vi "Goalie.vi"(3 "Defensores":u32[](array[numeric]), 5 "AI Parameters":T1={"GotoKick"={"Dist do cone a frente"=150.0, "attacker farback"=1500.0, "Perto"=300.0, "min dist to kick"=150.0, "kick eps"=0.0, "Time to transition"=0.05}, "Attacker"={"CC chute"=0.09, "CC passe"=0.045, "Kick Force"=100.0, "D ball-robot Kick"=200.0, "D ball-robot Pass"=0.3}, "Defender"={"D max"=1700.0, "Vel p/ robô av"=1000.0, "Kick Force"=100.0, "D atk-def"=0.0, "D farback"=0.0}, "Timeout"={"Field/v in x"=6.0, "Dist Robots"=300, "Dist up in y"=300}, "Pose Striker"={"dist"=200.0, "Numeric"=-4.0, "dist 2"=200.0}, "Dist Stop"=300.0, "Distance when ball out"=200, "D central gap "=150.0, "T pass"=0.0, "Force ++"=0.0, "range kick"=0.0, "Chute alto"=TRUE, "Marcador novo"=TRUE} {"D central gap" format="%#_13g"; "Dist Stop" format="%#_13g"; "Pose Striker"."Numeric" format="%#_13g"; "Defender"."Kick Force" format="%#_13g"; "Defender"."Vel p/ robô av" format="%#_13g"; "Attacker"."D ball-robot Kick" format="%#_13g"; "Attacker"."Kick Force" format="%#_13g"; "Attacker"."CC passe" format="%#_13g"; "Attacker"."CC chute" format="%#_13g"; "GotoKick"."kick eps" format="%#_13g"; "GotoKick"."min dist to kick" format="%#_13g"; "GotoKick"."Perto" format="%#_13g"; "GotoKick"."attacker farback" format="%#_13g"; "GotoKick"."Dist do cone a frente" format="%#_13g"}, 7 "Total de robos":u32[](array[numeric]), 8 "Field defense":dbl[](array[numeric]), 9 "IA Input":T5={"our_robots"=[], "enemy_robots"=[], "balls"=[], "geometry"={"line_width"=0, "field_length"=0, "field_width"=0, "boundary_width"=0, "referee_width"=0, "goal_width"=0, "goal_depth"=0, "goal_wall_width"=0, "center_circle_radius"=0, "defense_radius"=0, "defense_stretch"=0, "free_kick_from_defense_dist"=0, "penalty_spot_from_field_line_dist"=0, "penalty_line_from_spot_dist"=0}, "IA Judge"={"stage"="", "command"="", "our_goalie_id"=0.0, "enemy_goalie_id"=0.0, "command enum"=enum."Halt", "Time"=enum."Azul"}, "Received Timestamp"=timestamp(0 s since 1904-01-01), "Events"={"Touch"=FALSE, "Ball out"=FALSE, "id touch"=0.0, "Ball out of \nVision"=FALSE, "Ball inside \nGoalie area"=FALSE, "Robot not responding"=FALSE, "Robots responding status"=[1.0, 1.0, 1.0, 1.0, 1.0, 1.0], "Enemy Ball \nPossession"=FALSE, "Pass State"=FALSE, "id end of pass"=0.0, "Kick"=FALSE, "Id ini Possession"=0.0, "Ball Possesion"=FALSE, "Id Possesion"=0.0}}, 10 "Robot":T2={"id"=0, "function"=enum."Attacker", "x"=0.0, "y"=0.0, "orientation"=0.0, "v_tangent"=0.0, "v_normal"=0.0, "v_ang"=0.0, "kick_x"=0.0, "kick_z"=0.0, "dribble"=FALSE, "Timestamp"=timestamp(0 s since 1904-01-01), "dest_x"=0.0, "dest_y"=0.0, "dest_orientation"=0.0, "estimatives"={"est_v_tangent"=0.0, "est_v_normal"=0.0, "est_vx"=0.0, "est_vy"=0.0, "Pos Robot Est"=[]}, "dest_x_kick"=0.0, "dest_y_kick"=0.0, "Gap Coord"=[], "States"=enum."GoToTangent"}, 11 "command\nenum":T9) -> (2 "output cluster":T2={"id"=0, "function"=enum."Attacker", "x"=0.0, "y"=0.0, "orientation"=0.0, "v_tangent"=0.0, "v_normal"=0.0, "v_ang"=0.0, "kick_x"=0.0, "kick_z"=0.0, "dribble"=FALSE, "Timestamp"=timestamp(0 s since 1904-01-01), "dest_x"=0.0, "dest_y"=0.0, "dest_orientation"=0.0, "estimatives"={"est_v_tangent"=0.0, "est_v_normal"=0.0, "est_vx"=0.0, "est_vy"=0.0, "Pos Robot Est"=[]}, "dest_x_kick"=0.0, "dest_y_kick"=0.0, "Gap Coord"=[], "States"=enum."GoToTangent"})   [LabVIEW 2016]
uses:
  Core/AI Robot.ctl
  Functions Enum.ctl
  AttackerStates.ctl
  Command Enum.ctl
  Core/AI Input.ctl
  Core/AI Ball.ctl
  Core/Field Size.ctl
  Core/AI Judge.ctl
  Util/Events/Events.ctl
  AI Parameters.ctl
  <vilib>/Analysis/NI_AALPro.lvlib
  <vilib>/Analysis/_algsub.llb/Real Vector Norm.vi
panel:
  in  "y":dbl=100.0 format="%#_13g"
  out "Modulo":dbl
  in  "Time kick (s)":dbl=1.0 caption="Time Target (s)"
  in  "min dist to kick 2":dbl=112.0 format="%#_13g"
  in  "attck contra?":dbl
  in  "min dist to kick":dbl=195.0 format="%#_13g"
  in  "T":dbl[](array[numeric])
  in  "Vel min":dbl=10.0 format="%#_13g"
  in  "Attacker Distance":dbl=200.0
  out "Closest Robot":T2={"id"=0, "function"=enum."Attacker", "x"=0.0, "y"=0.0, "orientation"=0.0, "v_tangent"=0.0, "v_normal"=0.0, "v_ang"=0.0, "kick_x"=0.0, "kick_z"=0.0, "dribble"=FALSE, "Timestamp"=timestamp(0 s since 1904-01-01), "dest_x"=0.0, "dest_y"=0.0, "dest_orientation"=0.0, "estimatives"={"est_v_tangent"=0.0, "est_v_normal"=0.0, "est_vx"=0.0, "est_vy"=0.0, "Pos Robot Est"=[]}, "dest_x_kick"=0.0, "dest_y_kick"=0.0, "Gap Coord"=[], "States"=enum."GoToTangent"}
  out "Max Dist":dbl=999999999.0 format="%#_13g"
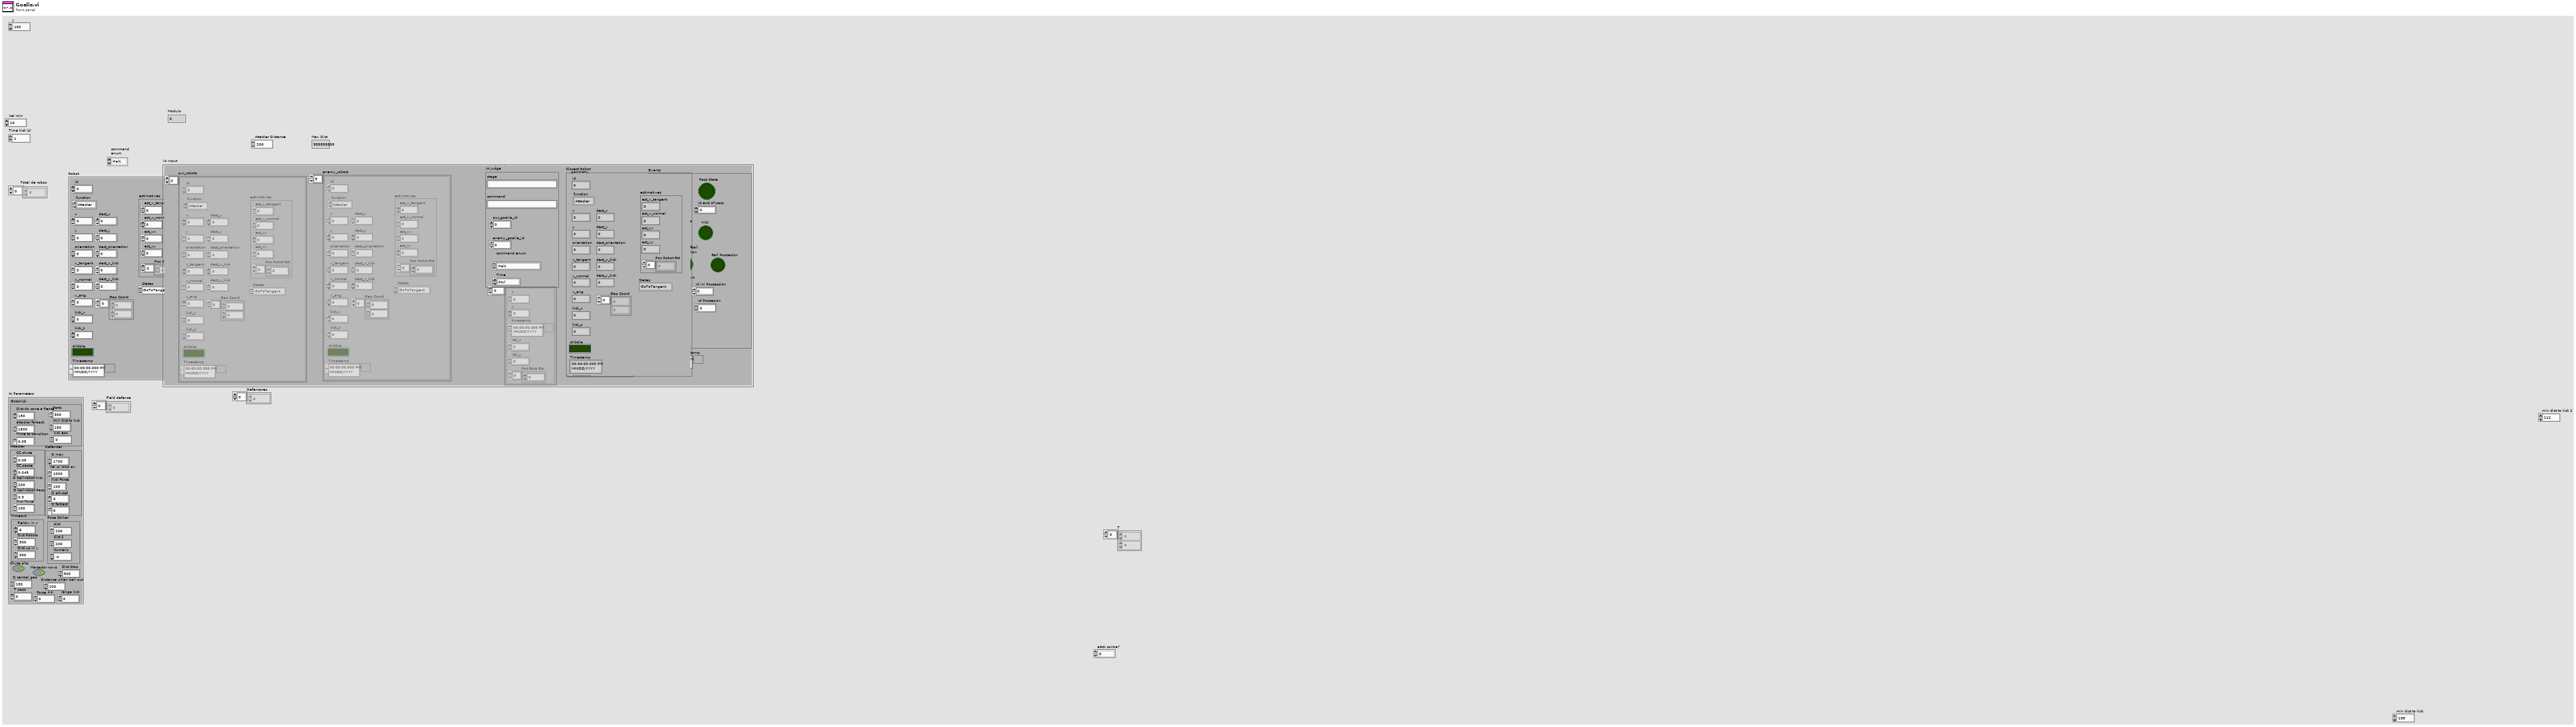
[diagram p1: front panel]
types:
  T1 = typedef "AI Parameters.ctl" = cluster{"GotoKick":cluster{"Dist do cone a frente":dbl, "attacker farback":dbl, "Perto":dbl, "min dist to kick":dbl, "kick eps":dbl, "Time to transition":dbl}, "Attacker":cluster{"CC chute":dbl, "CC passe":dbl, "Kick Force":dbl, "D ball-robot Kick":dbl, "D ball-robot Pass":dbl}, "Defender":cluster{"D max":dbl, "Vel p/ robô av":dbl, "Kick Force":dbl, "D atk-def":dbl, "D farback":dbl}, "Timeout":cluster{"Field/v in x":dbl, "Dist Robots":u32, "Dist up in y":u32}, "Pose Striker":cluster{"dist":dbl, "Numeric":dbl, "dist 2":dbl}, "Dist Stop":dbl, "Distance when ball out":i32, "D central gap ":dbl, "T pass":dbl, "Force ++":dbl, "range kick":dbl, "Chute alto":bool, "Marcador novo":bool}
  T2 = typedef "AI Robot.ctl" = cluster{"id":u32, "function":T3, "x":dbl, "y":dbl, "orientation":dbl, "v_tangent":dbl, "v_normal":dbl, "v_ang":dbl, "kick_x":dbl, "kick_z":dbl, "dribble":bool, "Timestamp":timestamp, "dest_x":dbl, "dest_y":dbl, "dest_orientation":dbl, "estimatives":cluster{"est_v_tangent":dbl, "est_v_normal":dbl, "est_vx":dbl, "est_vy":dbl, "Pos Robot Est":dbl[]}, "dest_x_kick":dbl, "dest_y_kick":dbl, "Gap Coord":dbl[], "States":T4}
  T3 = typedef "Functions Enum.ctl" = enum16{"Attacker", "Goalie", "Defender", "Striker", "Goto 0", "Dummy", "Kicker", "ZigZag"}
  T4 = typedef "AttackerStates.ctl" = enum16{"Pass", "GoToTangent", "BallGetting", "GoToKick", ""}
  T5 = typedef "AI Input.ctl" = cluster{"our_robots":T2[], "enemy_robots":T2[], "balls":T6[], "geometry":T7, "IA Judge":T8, "Received Timestamp":timestamp, "Events":T10}
  T6 = typedef "AI Ball.ctl" = cluster{"x":dbl, "y":dbl, "timestamp":timestamp, "Vel_x":dbl, "Vel_y":dbl, "Pos Bola Est":dbl[]}
  T7 = typedef "Field Size.ctl" = cluster{"line_width":u32, "field_length":u32, "field_width":u32, "boundary_width":u32, "referee_width":u32, "goal_width":u32, "goal_depth":u32, "goal_wall_width":u32, "center_circle_radius":u32, "defense_radius":u32, "defense_stretch":u32, "free_kick_from_defense_dist":u32, "penalty_spot_from_field_line_dist":u32, "penalty_line_from_spot_dist":u32}
  T8 = typedef "AI Judge.ctl" = cluster{"stage":string, "command":string, "our_goalie_id":dbl, "enemy_goalie_id":dbl, "command enum":T9, "Time":enum16{"Azul", "Amarelo"}}
  T9 = typedef "Command Enum.ctl" = enum16{"Halt", "Stop", "Force Start", "PKA Normal Start", "Prepare Kickoff Ally", "PKE Normal Start", "Prepare Kickoff Enemy", "Prepare Penalty Ally", "PPA Normal Start", "Prepare Penalty Enemy", "PPE Normal Start", "Direct Free Enemy", "Direct Free Ally", "Indirect Free Enemy", "Indirect Free Ally", "Timeout Enemy", "Timeout Ally", "Goal Enemy", "Goal Ally", "Ball Placement Enemy", "Ball Placement Ally", "Normal Half Time", "Extra Time Break", "Extra Half Time", "None", "Post Game"}
  T10 = typedef "Events.ctl" = cluster{"Touch":bool, "Ball out":bool, "id touch":dbl, "Ball out of \nVision":bool, "Ball inside \nGoalie area":bool, "Robot not responding":bool, "Robots responding status":dbl[], "Enemy Ball \nPossession":bool, "Pass State":bool, "id end of pass":dbl, "Kick":bool, "Id ini Possession":dbl, "Ball Possesion":bool, "Id Possesion":dbl}
  T11 = typedef "AI Robot.ctl" = cluster{"id":u32, "function":T12, "x":dbl, "y":dbl, "orientation":dbl, "v_tangent":dbl, "v_normal":dbl, "v_ang":dbl, "kick_x":dbl, "kick_z":dbl, "dribble":bool, "Timestamp":timestamp, "dest_x":dbl, "dest_y":dbl, "dest_orientation":dbl}
  T12 = typedef "Functions Enum.ctl" = enum16{"Attacker", "Goalie", "Defender", "Goto 0", "Dummy", "ZigZag"}
  T13 = typedef "AI Robot.ctl" = cluster{"id":u32, "function":T3, "x":dbl, "y":dbl, "orientation":dbl, "v_tangent":dbl, "v_normal":dbl, "v_ang":dbl, "kick_x":dbl, "kick_z":dbl, "dribble":bool, "Timestamp":timestamp, "dest_x":dbl, "dest_y":dbl, "dest_orientation":dbl, "estimatives":cluster{"est_v_tangent":dbl, "est_v_normal":dbl, "est_vx":dbl, "est_vy":dbl}, "dest_x_kick":dbl, "dest_y_kick":dbl, "Gap Coord":dbl[], "States":T4}
  T14 = typedef "AI Ball.ctl" = cluster{"x":dbl, "y":dbl, "timestamp":timestamp, "Vel_x":dbl, "Vel_y":dbl}
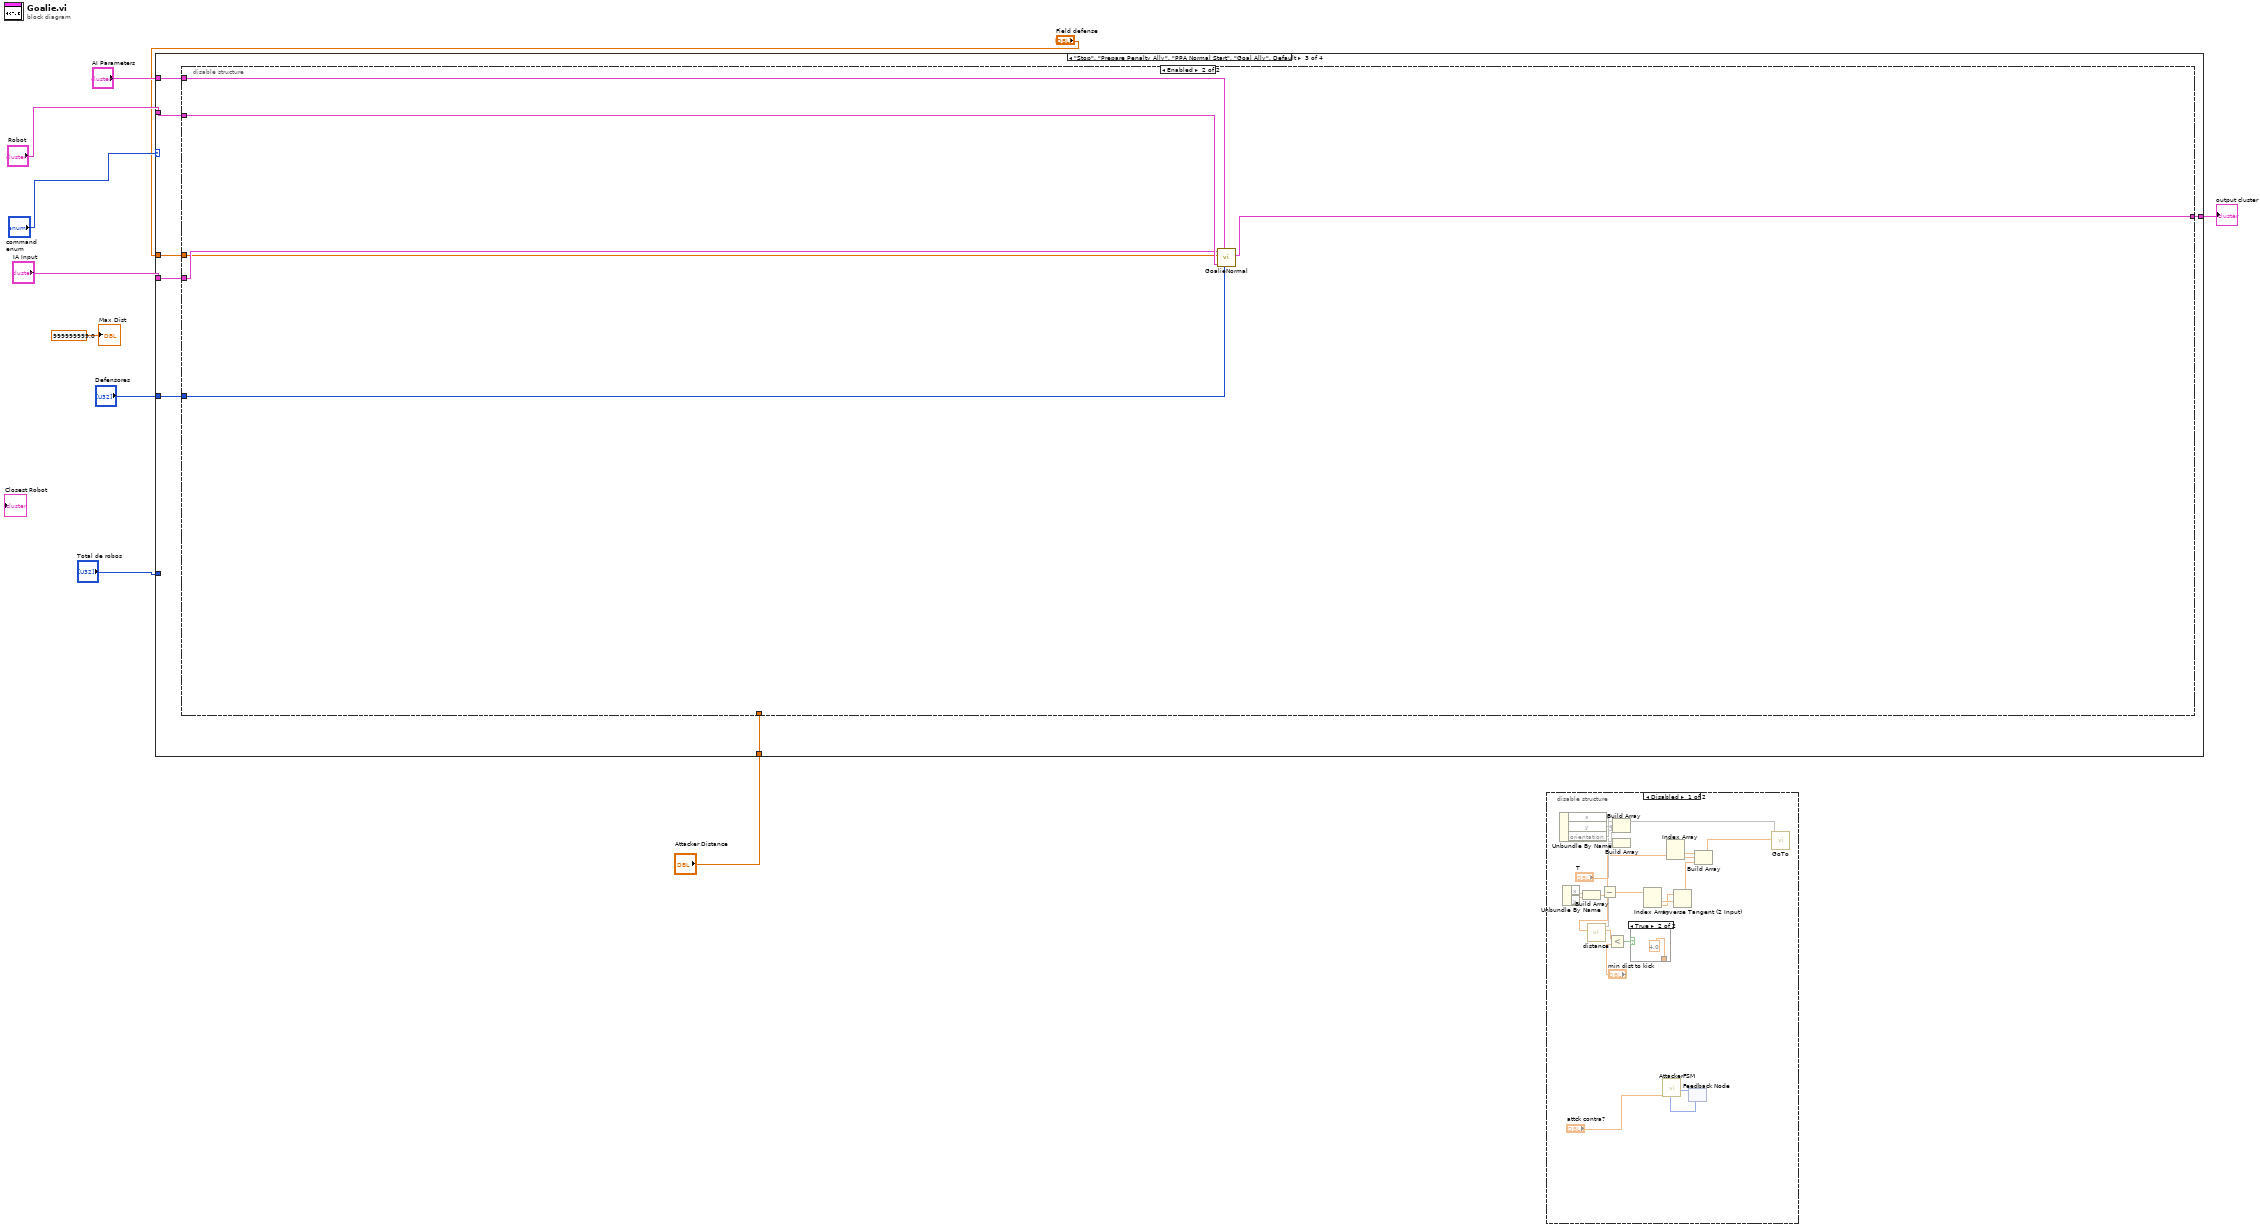
[diagram p0: block diagram]
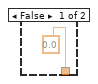
[diagram p2: hidden frame]
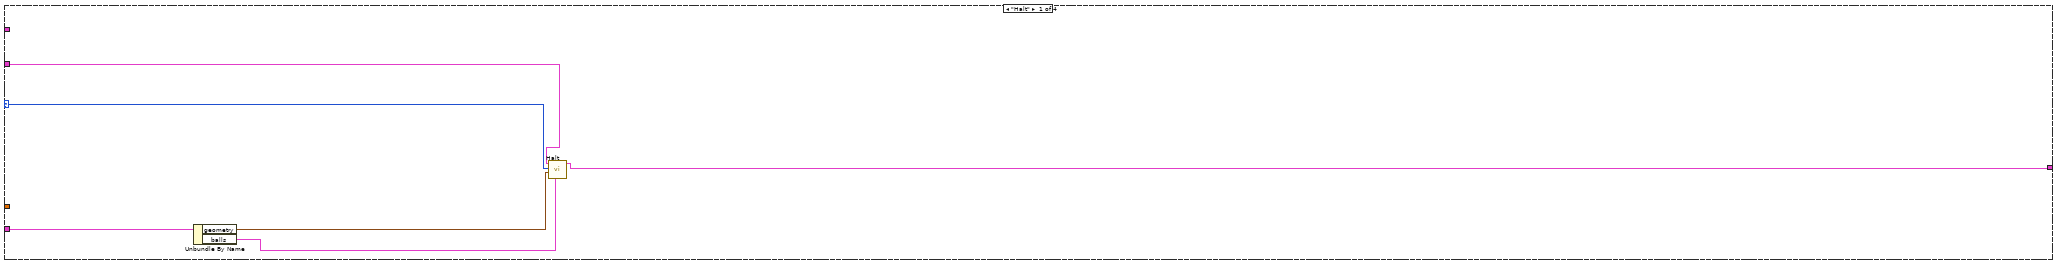
[diagram p4: hidden frame]
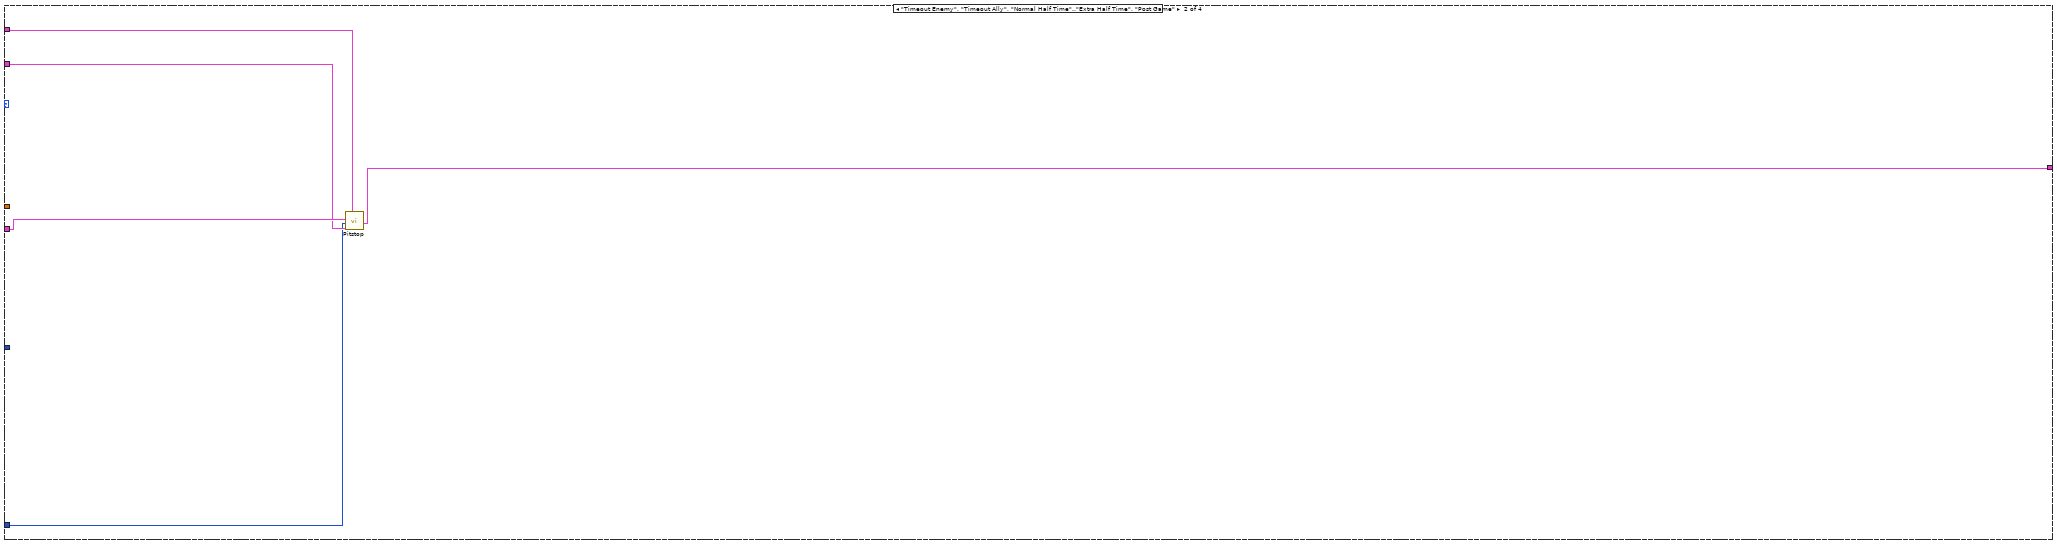
[diagram p5: hidden frame]
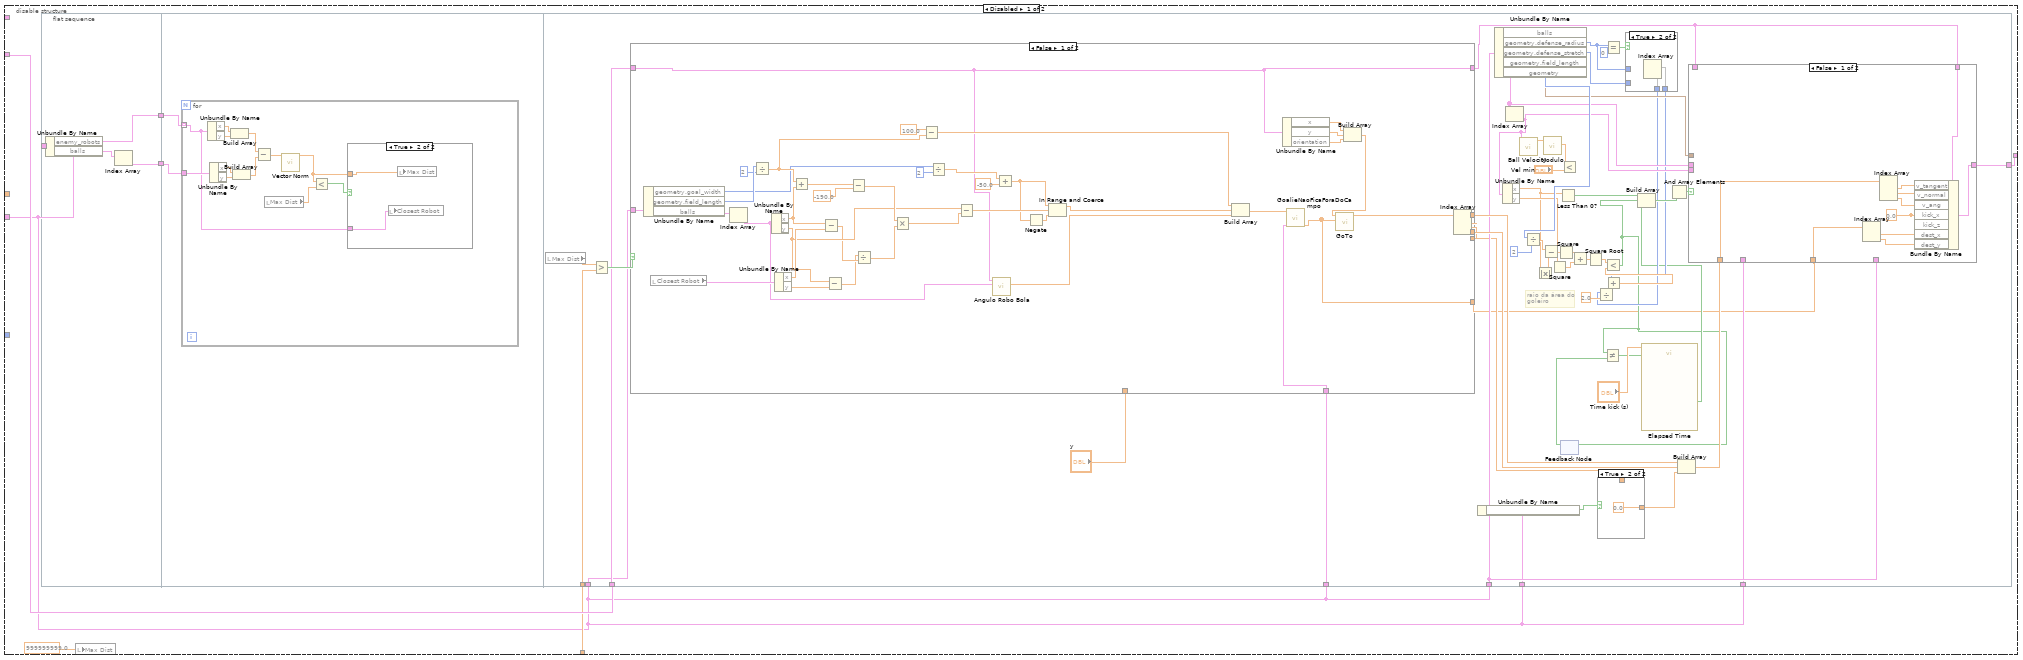
[diagram p6: hidden frame]
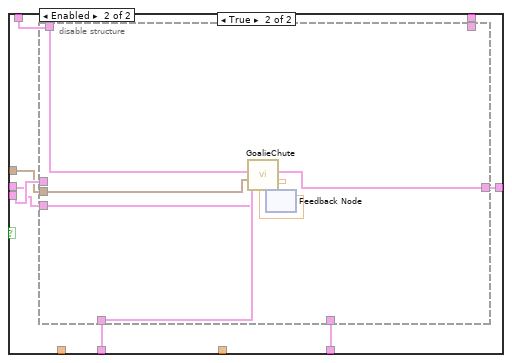
[diagram p10: hidden frame]
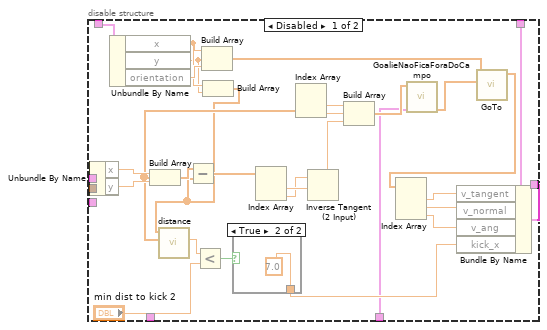
[diagram p11: hidden frame]
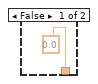
[diagram p12: hidden frame]
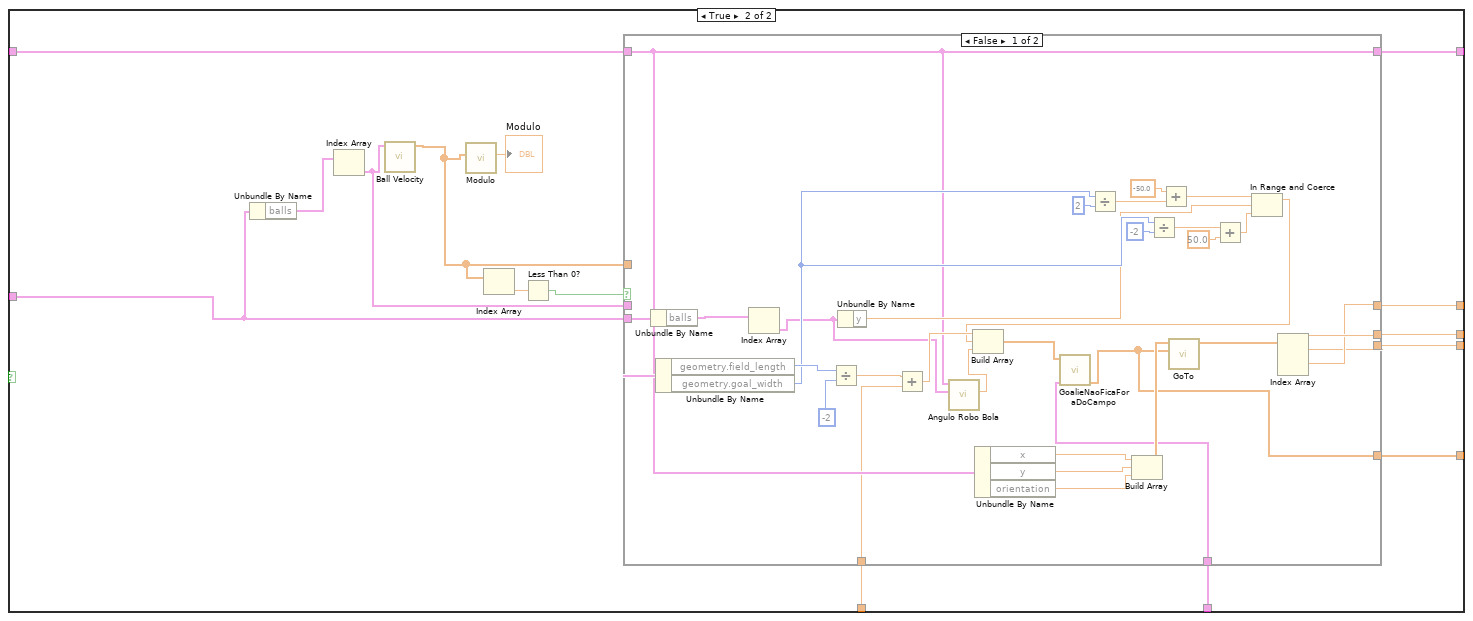
[diagram p13: hidden frame]
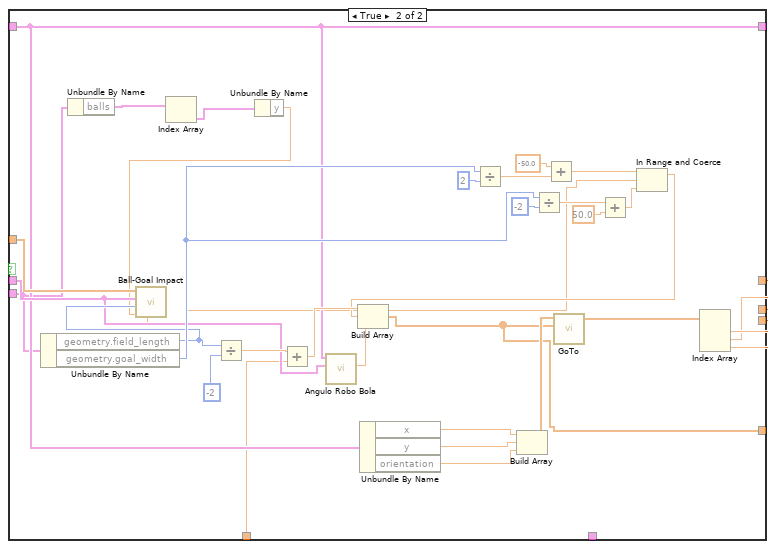
[diagram p14: hidden frame]
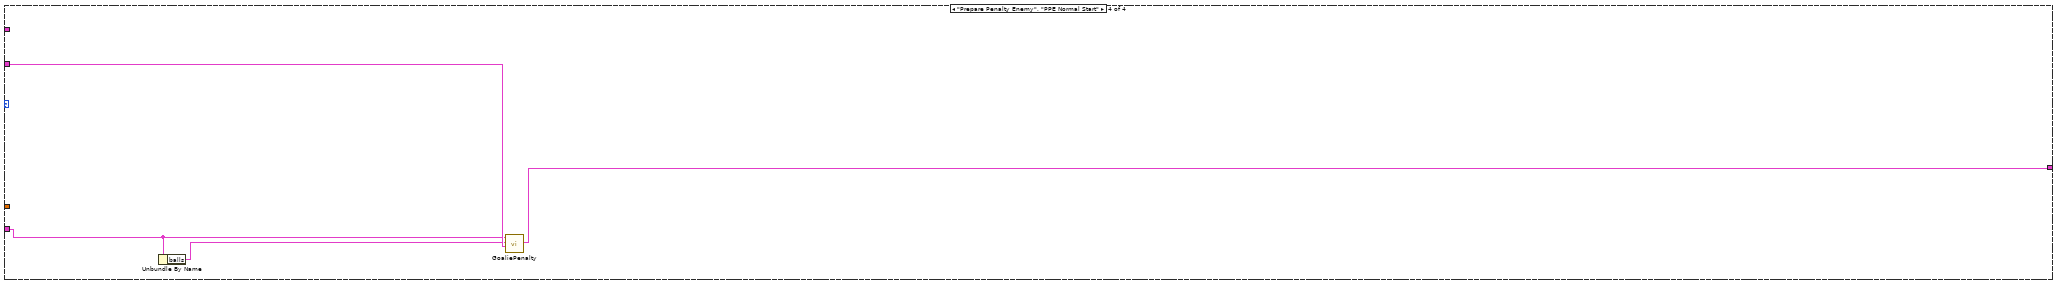
[diagram p15: hidden frame]
diagram:
  n1 = case shown="\"Stop\", \"Prepare Penalty Ally\", \"PPA Normal Start\", \"Goal Ally\", Default" "command\nenum" {
    selector: "command\nenum" -> [w11 _ _ _]
    tunnel: "Robot" -> [w16 w20 w28 w301]
    tunnel: [w15 w19 w26 w298] -> w7
    tunnel: "IA Input" -> [w14 w21 w25 w300]
    tunnel: "Attacker Distance" -> [_ _ w27 _]
    tunnel: "Total de robos" -> [_ w18 _ _]
    tunnel: "AI Parameters" -> [_ w17 w24 _]
    tunnel: "Field defense" -> [_ _ w23 _]
    tunnel: "Defensores" -> [_ _ w22 _]
    frame "Halt" {
      n2 = Unbundle By Name(w14) -> ("geometry"=w12:T7, "balls"=w13:T6[])
      n3 = call "Halt.vi"("balls"=w13, "Field Size in"=w12, "Numeric"=w11, "Robot in"=w16) -> ("Robot out"=w15:T2)  [unwired: 7 in]
    }
    frame "Timeout Enemy", "Timeout Ally", "Normal Half Time".."Extra Half Time", "Post Game" {
      n4 = call "Pitstop.vi"("AI Parameters"=w17, "Robot in"=w20, "robos"=w18, "IA State Input"=w21) -> ("Robot out"=w19:T2)  [unwired: 7 in]
    }
    frame "Stop", "Prepare Penalty Ally", "PPA Normal Start", "Goal Ally", Default {
      n5 = disable-structure shown="Enabled" {
        disable-tunnel: w28 -> [w33 w297]
        disable-tunnel: w27 -> [w32 _]
        disable-tunnel: [w30 w295] -> w26
        disable-tunnel: w25 -> [w29 w296]
        disable-tunnel: w24 -> [_ w294]
        disable-tunnel: w23 -> [_ w293]
        disable-tunnel: w22 -> [_ w292]
        frame Disabled {
          n6 = flat-sequence {
            tunnel: w29 -> [w39]
            tunnel: [w38] -> w35
            tunnel: [w36] -> w34
            tunnel: w35 -> [w41]
            tunnel: w34 -> [w40]
            tunnel: w33 -> [w106]
            tunnel: w29 -> [w105]
            tunnel: w32 -> [w104]
            tunnel: w29 -> [w69]
            tunnel: [w78] -> w30
            tunnel: w29 -> [w68]
            tunnel: w29 -> [w67]
            tunnel: w29 -> [w61]
            frame #0 {
              n7 = Unbundle By Name(w39) -> ("enemy_robots"=w38:T2[], "balls"=w37:T6[])
              n8 = Index Array(array=w37) -> (element=w36:T6)  [unwired: 1 in]
            }
            frame #1 {
              n9 = for {
                tunnel: w41 -> [w43] mode=indexing
                tunnel: w40 -> [w53]
                n10 = Unbundle By Name(w43) -> ("x"=w52:dbl, "y"=w51:dbl)
                n11 = Unbundle By Name(w53) -> ("x"=w50:dbl, "y"=w49:dbl)
                n12 = Build Array(w52, w51) -> (w48:dbl[])
                n13 = Build Array(w50, w49) -> (w47:dbl[])
                n14 = Subtract(x=w48, y=w47) -> (x-y=w46:dbl[])
                n15 = local read "Max Dist"() -> (w45:dbl)
                n16 = call-poly <vilib>:"Vector Norm.vi"("Input Vector"=w46) -> ("norm"=w42:dbl)  [unwired: 9 in, 1 out]
                n17 = Less?(x=w42, y=w45) -> (x < y?=w44:bool)
                n18 = case shown="True" w44 {
                  tunnel: w43 -> [_ w55]
                  tunnel: w42 -> [_ w54]
                  frame False {
                  }
                  frame True {
                    n19 = local write "Closest Robot"(w55) -> ()
                    n20 = local write "Max Dist"(w54) -> ()
                  }
                }
              }
            }
            frame #2 {
              # "raio da área do \ngoleiro"
              n21 = local read "Max Dist"() -> (w107:dbl)
              n22 = Greater?(x=w107, y=w104) -> (0:w108:bool)
              n23 = case shown="False" w108 {
                tunnel: w106 -> [w174 w226]
                tunnel: w105 -> [w211 w225]
                tunnel: [w177 w222] -> w101
                tunnel: [w176 w221] -> w99
                tunnel: [w175 w220] -> w58
                tunnel: [w174 w219] -> w77
                tunnel: w68 -> [w172 w218]
                tunnel: "y" -> [_ w213]
                tunnel: [w171 w212] -> w56
                frame False {
                  n24 = Unbundle By Name(w211) -> ("geometry.goal_width"=w186:u32, "geometry.field_length"=w207:u32, "balls"=w210:T6[])
                  n25 = local read "Closest Robot"() -> (w209:T2)
                  n26 = Index Array(array=w210) -> (element=w179:T6)  [unwired: 1 in]
                  n27 = Divide(x=w207, y=u32 2) -> (x/y=w196:dbl)
                  n28 = Unbundle By Name(w179) -> ("x"=w205:dbl, "y"=w199:dbl)
                  n29 = Unbundle By Name(w209) -> ("x"=w208:dbl, "y"=w198:dbl)
                  n30 = Add(x=w196, y=w205) -> (x+y=w204:dbl)
                  n31 = Subtract(x=w205, y=w208) -> (x-y=w189:dbl)
                  n32 = Subtract(x=w199, y=w198) -> (x-y=w188:dbl)
                  n33 = Subtract(x=w204, y=-190.0) -> (x-y=w202:dbl)
                  n34 = Divide(x=w188, y=w189) -> (x/y=w201:dbl)
                  n35 = Multiply(x=w202, y=w201) -> (x*y=w200:dbl)
                  n36 = Subtract(x=100.0, y=w196) -> (x-y=w195:dbl)
                  n37 = Divide(x=w186, y=u32 2) -> (x/y=w184:dbl)
                  n38 = Subtract(x=w199, y=w200) -> (x-y=w187:dbl)
                  n39 = call "Angulo Robo Bola.vi"("Ball"=w179, "Robot"=w174) -> ("Angulo"=w178:dbl)  [unwired: 9 in]
                  n40 = Add(x=w184, y=-50.0) -> (x+y=w181:dbl)
                  n41 = Negate(x=w181) -> (-x=w182:dbl)
                  n42 = In Range and Coerce(upper limit=w181, x=w187, lower limit=w182) -> (coerced(x)=w180:dbl)  [unwired: 1 out]
                  n43 = Build Array(w195, w180, w178) -> (w173:dbl[])
                  n44 = Unbundle By Name(w174) -> ("x"=w194:dbl, "y"=w193:dbl, "orientation"=w192:dbl)
                  n45 = call "GoalieNaoFicaForaDoCampo.vi"("IA Input"=w172, "PositionIn"=w173) -> ("PositionOut"=w171:dbl[])  [unwired: 9 in]
                  n46 = Build Array(w194, w193, w192) -> (w191:dbl[])
                  n47 = call "GoTo.vi"("Target"=w171, "Position"=w191) -> ("Output\nVelocity"=w190:dbl[])  [unwired: 8 in, 1 out]
                  n48 = Index Array(array=w190) -> (element #1=w177:dbl, element #2=w176:dbl, element #3=w175:dbl)  [unwired: 3 in]
                }
                frame True {
                  n49 = Unbundle By Name(w225) -> ("balls"=w224:T6[])
                  n50 = Index Array(array=w224) -> (element=w223:T6)  [unwired: 1 in]
                  n51 = call "Ball Velocity.vi"("Ball"=w223) -> ("Velocity"=w216:dbl[])  [unwired: 10 in]
                  n52 = call "Modulo.vi"("2D vector"=w216) -> ("Modulo"=→"Modulo":dbl)  [unwired: 10 in]
                  n53 = Index Array(array=w216) -> (element=w215:dbl)  [unwired: 1 in]
                  n54 = Less Than 0?(x=w215) -> (x < 0?=w214:bool)
                  n55 = case shown="False" w214 {
                    tunnel: w225 -> [w254 w263]
                    tunnel: w226 -> [w234 w266]
                    tunnel: w216 -> [_ w272]
                    tunnel: w223 -> [_ w271]
                    tunnel: [w233 w269] -> w222
                    tunnel: [w232 w268] -> w221
                    tunnel: [w231 w267] -> w220
                    tunnel: [w234 w266] -> w219
                    tunnel: w218 -> [w229 _]
                    tunnel: w213 -> [w228 w262]
                    tunnel: [w227 w259] -> w212
                    frame False {
                      n56 = Unbundle By Name(w254) -> ("balls"=w253:T6[])
                      n57 = Unbundle By Name(w254) -> ("geometry.field_length"=w252:u32, "geometry.goal_width"=w247:u32)
                      n58 = Index Array(array=w253) -> (element=w236:T6)  [unwired: 1 in]
                      n59 = Divide(x=w252, y=-2) -> (x/y=w251:dbl)
                      n60 = Unbundle By Name(w236) -> ("y"=w243:dbl)
                      n61 = Add(x=w251, y=w228) -> (x+y=w250:dbl)
                      n62 = call "Angulo Robo Bola.vi"("Ball"=w236, "Robot"=w234) -> ("Angulo"=w235:dbl)  [unwired: 9 in]
                      n63 = Unbundle By Name(w234) -> ("x"=w256:dbl, "y"=w258:dbl, "orientation"=w257:dbl)
                      n64 = Divide(x=w247, y=2) -> (x/y=w240:dbl)
                      n65 = Build Array(w256, w258, w257) -> (w249:dbl[])
                      n66 = Divide(x=w247, y=-2) -> (x/y=w242:dbl)
                      n67 = Add(x=-50.0, y=w240) -> (x+y=w238:dbl)
                      n68 = Add(x=w242, y=50.0) -> (x+y=w237:dbl)
                      n69 = In Range and Coerce(upper limit=w238, x=w243, lower limit=w237) -> (coerced(x)=w244:dbl)  [unwired: 1 out]
                      n70 = Build Array(w250, w244, w235) -> (w230:dbl[])
                      n71 = call "GoalieNaoFicaForaDoCampo.vi"("IA Input"=w229, "PositionIn"=w230) -> ("PositionOut"=w227:dbl[])  [unwired: 9 in]
                      n72 = call "GoTo.vi"("Target"=w227, "Position"=w249) -> ("Output\nVelocity"=w248:dbl[])  [unwired: 8 in, 1 out]
                      n73 = Index Array(array=w248) -> (element #1=w233:dbl, element #2=w232:dbl, element #3=w231:dbl)  [unwired: 3 in]
                    }
                    frame True {
                      n74 = Unbundle By Name(w263) -> ("geometry.field_length"=w273:u32, "geometry.goal_width"=w283:u32)
                      n75 = Unbundle By Name(w263) -> ("balls"=w265:T6[])
                      n76 = Index Array(array=w265) -> (element=w264:T6)  [unwired: 1 in]
                      n77 = Divide(x=w273, y=-2) -> (x/y=w287:dbl)
                      n78 = Unbundle By Name(w264) -> ("y"=w260:dbl)
                      n79 = call "Ball-Goal Impact.vi"("y"=w260, "Field Length"=w273, "Ball"=w271, "Ball Velocity"=w272) -> ("Y Collision"=w261:dbl)  [unwired: 7 in]
                      n80 = Add(x=w287, y=w262) -> (x+y=w286:dbl)
                      n81 = call "Angulo Robo Bola.vi"("Ball"=w271, "Robot"=w266) -> ("Angulo"=w270:dbl)  [unwired: 9 in]
                      n82 = Unbundle By Name(w266) -> ("x"=w289:dbl, "y"=w291:dbl, "orientation"=w290:dbl)
                      n83 = Divide(x=w283, y=2) -> (x/y=w277:dbl)
                      n84 = Build Array(w289, w291, w290) -> (w285:dbl[])
                      n85 = Divide(x=w283, y=-2) -> (x/y=w279:dbl)
                      n86 = Add(x=-50.0, y=w277) -> (x+y=w275:dbl)
                      n87 = Add(x=w279, y=50.0) -> (x+y=w274:dbl)
                      n88 = In Range and Coerce(upper limit=w275, x=w261, lower limit=w274) -> (coerced(x)=w280:dbl)  [unwired: 1 out]
                      n89 = Build Array(w286, w280, w270) -> (w259:dbl[])
                      n90 = call "GoTo.vi"("Target"=w259, "Position"=w285) -> ("Output\nVelocity"=w284:dbl[])  [unwired: 8 in, 1 out]
                      n91 = Index Array(array=w284) -> (element #1=w269:dbl, element #2=w268:dbl, element #3=w267:dbl)  [unwired: 3 in]
                    }
                  }
                }
              }
              n92 = Unbundle By Name(w61) -> ("Events.Ball inside \nGoalie area"=w60:bool)
              n93 = Unbundle By Name(w69) -> ("balls"=w80:T6[], "geometry.defense_radius"=w71:u32, "geometry.defense_stretch"=w70:u32, "geometry.field_length"=w87:u32, "geometry"=w79:T7)
              n94 = Index Array(array=w80) -> (element=w76:T6)  [unwired: 1 in]
              n95 = Unbundle By Name(w76) -> ("x"=w82:dbl, "y"=w85:dbl)
              n96 = call "Ball Velocity.vi"("Ball"=w76) -> ("Velocity"=w103:dbl[])  [unwired: 10 in]
              n97 = Divide(x=w87, y=u32 2) -> (x/y=w88:dbl)
              n98 = Absolute Value(x=w82) -> (abs(x)=w81:dbl)
              n99 = Subtract(x=w88, y=w81) -> (x-y=w94:dbl)
              n100 = call "Modulo.vi"("2D vector"=w103) -> ("Modulo"=w102:dbl)  [unwired: 10 in]
              n101 = Square(x=w85) -> (x^2=w93:dbl)
              n102 = Square(x=w94) -> (x^2=w92:dbl)
              n103 = Less Than 0?(x=w82) -> (x < 0?=w95:bool)
              n104 = feedback #1() -> (w62:bool)  [unwired: 1 in]
              n105 = Less?(x=w102, y="Vel min") -> ()  [unwired: 1 out]
              n106 = Add(x=w92, y=w93) -> (x+y=w83:dbl)
              n107 = Square Root(x=w83) -> (sqrt(x)=w84:dbl)
              n108 = case shown="True" w60 {
                tunnel: [w109 0.0] -> w59
                tunnel: w58 -> [w109 _]
                frame False {
                }
                frame True {
                }
              }
              n109 = Equal?(x=w71, y=u32 0) -> (x = y?=w74:bool)
              n110 = case shown="True" w74 {
                tunnel: [w112 w114] -> w73
                tunnel: [w111 w113] -> w72
                tunnel: w71 -> [w112 _]
                tunnel: w70 -> [w111 _]
                frame False {
                }
                frame True {
                  n111 = Index Array() -> (element #1=w114, element #2=w113)  [unwired: 3 in]
                }
              }
              n112 = Divide(x=w72, y=2.0) -> (x/y=w91:dbl)
              n113 = Add(x=w73, y=w91) -> (x+y=w89:dbl)
              n114 = Less?(x=w84, y=w89) -> (x < y?=w63:bool)
              n115 = feedback-in #1(w63) -> ()
              n116 = Not Equal?(x=w63, y=w62) -> (x != y?=w64:bool)
              n117 = call "Elapsed Time"("Time Target (s)"="Time kick (s)", "Reset"=w64) -> ("Time has Elapsed"=w65:bool)  [unwired: 10 in, 7 out]
              n118 = Build Array(w95, w63, w65) -> (w98:bool[])
              n119 = And Array Elements(Boolean array=w98) -> (logical AND=w97:bool)
              n120 = Build Array(w101, w99, w59) -> (w100:dbl[])
              n121 = case shown="False" w97 {
                tunnel: w80 -> [_ w125]
                tunnel: w77 -> [_ w132]
                tunnel: w100 -> [w119 _]
                tunnel: w79 -> [_ w126]
                tunnel: [w121 w130] -> w78
                tunnel: w77 -> [w120 w131]
                tunnel: w76 -> [_ w129]
                tunnel: w69 -> [_ w128]
                tunnel: w67 -> [_ w127]
                tunnel: w56 -> [w116 _]
                frame False {
                  w118 = 0.0
                  n122 = Index Array(array=w116) -> (element #1=w117:dbl, element #2=w115:dbl)  [unwired: 2 in]
                  n123 = Index Array(array=w119) -> (element #1=w124:dbl, element #2=w123:dbl, element #3=w122:dbl)  [unwired: 3 in]
                  n124 = Bundle By Name(cluster=w120, "v_tangent"=w124, "v_normal"=w123, "v_ang"=w122, "kick_x"=w118, "kick_z"=w118, "dest_x"=w117, "dest_y"=w115) -> (w121:T2)
                }
                frame True {
                  n125 = disable-structure shown="Enabled" {
                    disable-tunnel: w132 -> [w146 w169]
                    disable-tunnel: w131 -> [w141 _]
                    disable-tunnel: [w140 w164] -> w130
                    disable-tunnel: w129 -> [w138 _]
                    disable-tunnel: w128 -> [w134 _]
                    disable-tunnel: w127 -> [_ w170]
                    disable-tunnel: w126 -> [_ w168]
                    disable-tunnel: w125 -> [_ w167]
                    frame Disabled {
                      n126 = Unbundle By Name(w138) -> ("x"=w155:dbl, "y"=w154:dbl)
                      n127 = Unbundle By Name(w146) -> ("x"=w160:dbl, "y"=w159:dbl, "orientation"=w161:dbl)
                      n128 = Build Array(w155, w154) -> (w137:dbl[])
                      n129 = Build Array(w160, w159, w161) -> (w158:dbl[])
                      n130 = Build Array(w160, w159) -> (w136:dbl[])
                      n131 = call "distance.vi"("target pos"=w137, "obj pos"=w136) -> ("sqrt(x)"=w147:dbl)  [unwired: 9 in]
                      n132 = Subtract(x=w137, y=w136) -> (x-y=w153:dbl[])
                      n133 = Less?(x=w147, y="min dist to kick 2") -> (x < y?=w149:bool)
                      n134 = case shown="True" w149 {
                        tunnel: [0.0 7.0] -> w139
                        frame False {
                        }
                        frame True {
                        }
                      }
                      n135 = Index Array(array=w153) -> (element #1=w157:dbl, element #2=w156:dbl)  [unwired: 2 in]
                      n136 = Index Array(array=w137) -> (element #1=w151:dbl, element #2=w150:dbl)  [unwired: 2 in]
                      n137 = Inverse Tangent (2 Input)(1:w157, 2:w156) -> (0:w152:dbl)
                      n138 = Build Array(w151, w150, w152) -> (w135:dbl[])
                      n139 = call "GoalieNaoFicaForaDoCampo.vi"("IA Input"=w134, "PositionIn"=w135) -> ("PositionOut"=w133:dbl[])  [unwired: 9 in]
                      n140 = call "GoTo.vi"("Target"=w133, "Position"=w158) -> ("Output\nVelocity"=w142:dbl[])  [unwired: 8 in, 1 out]
                      n141 = Index Array(array=w142) -> (element #1=w143:dbl, element #2=w144:dbl, element #3=w145:dbl)  [unwired: 3 in]
                      n142 = Bundle By Name(cluster=w141, "v_tangent"=w143, "v_normal"=w144, "v_ang"=w145, "kick_x"=w139) -> (w140:T2)
                    }
                    frame Enabled {
                      n143 = feedback #2() -> (w165:dbl)  [unwired: 1 in]
                      n144 = call "GoalieChute.vi"("Current State"=w165, "balls"=w167, "Field Size in"=w168, "Robot in"=w169, "IA State Input 2"=w170) -> ("Next State"=w166:dbl, "Robot out"=w164:T2)  [unwired: 5 in]
                      n145 = feedback-in #2(w166) -> ()
                    }
                  }
                }
              }
            }
          }
          n146 = local write "Max Dist"(999999999.0 ("Max Dist")) -> ()
        }
        frame Enabled {
          n147 = call "GoalieNormal.vi"("Defensores"=w292, "AI Parameters"=w294, "Robot"=w297, "Field defense"=w293, "IA Input"=w296) -> ("output cluster"=w295:T2)  [unwired: 6 in]
        }
      }
    }
    frame "Prepare Penalty Enemy", "PPE Normal Start" {
      n148 = Unbundle By Name(w300) -> ("balls"=w299:T6[])
      n149 = call "GoaliePenalty.vi"("Robot in"=w301, "balls"=w299, "IA Input"=w300) -> ("Robot out"=w298:T2)  [unwired: 8 in]
    }
  }
  "output cluster" <- w7
  n150 = disable-structure shown="Disabled" {
    frame Disabled {
      n151 = Unbundle By Name() -> (w330:T11, "x"=w328, "y"=w327, "orientation"=w329)
      n152 = Unbundle By Name() -> ("x"=w323:dbl, "y"=w322:dbl)  [unwired: 1 in]
      n153 = Build Array(w323, w322) -> (w310:dbl[])
      n154 = Subtract(x="T", y=w310) -> (x-y=w320:dbl[])
      n155 = Build Array(w328, w327, w329) -> (w326:void[])
      n156 = Build Array(w328, w327) -> (w311:void[])
      n157 = call "distance.vi"("target pos"=w310, "obj pos"=w311) -> ("sqrt(x)"=w309:dbl)  [unwired: 9 in]
      n158 = Less?(x=w309, y="min dist to kick") -> (x < y?=w314:bool)
      n159 = case shown="True" w314 {
        tunnel: [0.0 4.0] -> w312
        frame False {
        }
        frame True {
        }
      }
      n160 = Index Array(array=w320) -> (element #1=w325:dbl, element #2=w324:dbl)  [unwired: 2 in]
      n161 = Index Array(array=w310) -> (element #1=w317:dbl, element #2=w316:dbl)  [unwired: 2 in]
      n162 = Inverse Tangent (2 Input)(1:w325, 2:w324) -> (0:w318:dbl)
      n163 = feedback #3() -> (w305:T4)  [unwired: 1 in]
      n164 = call "AttackerFSM.vi"("Current States"=w305, "atacando contra?"="attck contra?") -> ("Next State"=w304:T4, "Robot out"=w303:T13, "balls"=w306:T14[], "Field Size in"=w307:T7, "Robot in"=w308:T13)  [unwired: 5 in]
      n165 = feedback-in #3(w304) -> ()
      n166 = Build Array(w317, w316, w318) -> (w319:dbl[])
      n167 = call "GoTo.vi"("Target"=w319, "Position"=w326) -> ("Output\nVelocity"=w315:dbl[])  [unwired: 8 in, 1 out]
    }
    frame Enabled {
    }
  }
  "Max Dist" <- 999999999.0 ("Max Dist")
